vi "Helper - ToggleOverrides.vi"(7 "FocusObj":refnum<vi>, 8 "Rudder Override?":bool, 9 "Sail Override?":bool, 10 "VKey":T1=enum."Up", 11 "Char":i16) -> (1 "Override Rudder":bool, 2 "Override Sail":bool)   [LabVIEW 2011]
doc: "Takes in current values of sail and rudder override and togges them if the correct button is hit.\nOnly does something if you're actually looking at the OCU - use the event structure to get FocusObj.\n\nPotential problem: if you hit the button on the OCU and the keyboard button at the same time, they might end up cancelling each other out....\n\n-Elizabeth Mahon"
uses:
  <vilib>/event_ctls.llb/eventvkey.ctl
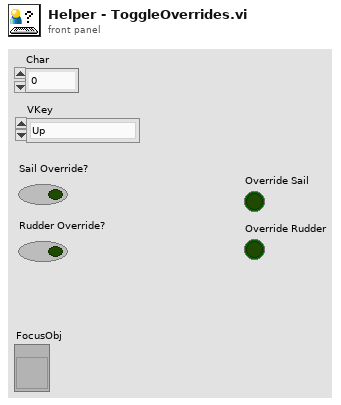
[diagram p1: front panel]
types:
  T1 = typedef "eventvkey.ctl" = enum16{"ASCII", "Enter", "Return", "Shift", "Ctrl", "Alt", "Cmd", "Opt", "Caps", "NumLock", "Clear", "Break", "Up", "Down", "Left", "Right", "Insert", "Delete", "Home", "End", "PageUp", "PageDown", "Escape", "Help", "Pause", "ScrollLock", "F1", "F2", "F3", "F4", "F5", "F6", "F7", "F8", "F9", "F10", "F11", "F12", "F13", "F14", "F15", "F16", "F17", "F18", "F19", "F20", "F21", "F22", "F23", "F24", "Play", "VolumeUp", "VolumeDown", "Mute", "Two Byte Char"}
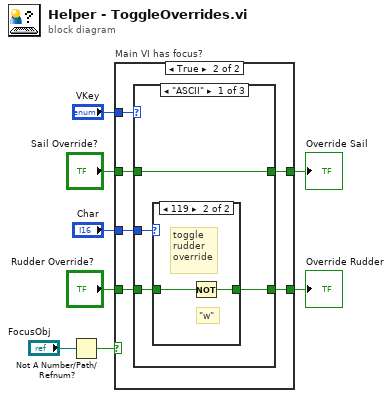
[diagram p0: block diagram]
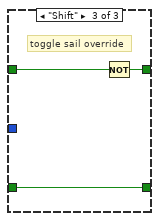
[diagram p5: hidden frame]
diagram:
  n1 = Not A Number/Path/Refnum?(number/path/refnum="FocusObj") -> (NaN/Path/Refnum?=w5:bool)
  n2 = case "Main VI has focus?" shown="True" w5 {
    tunnel: "VKey" -> [_ w16]
    tunnel: "Char" -> [_ w15]
    tunnel: "Sail Override?" -> [w10 w14]
    tunnel: [w10 w13] -> w3
    tunnel: "Rudder Override?" -> [w9 w12]
    tunnel: [w9 w11] -> w1
    frame False {
    }
    frame True {
      n3 = case shown="\"ASCII\"" w16 {
        tunnel: w15 -> [w20 _ _]
        tunnel: w14 -> [w19 w25 w27]
        tunnel: [w19 w25 w28] -> w13
        tunnel: w12 -> [w18 w24 w26]
        tunnel: [w17 w24 w26] -> w11
        frame "ASCII" {
          n4 = case shown="119" w20 {
            tunnel: w18 -> [w21 w23]
            tunnel: [w21 w22] -> w17
            frame 0, Default {
            }
            frame 119 {
              # "toggle\nrudder\noverride"
              # "\"w\""
              n5 = Not(x=w23) -> (.not. x?=w22:bool)
            }
          }
        }
        frame Default {
        }
        frame "Shift" {
          # "toggle sail override"
          n6 = Not(x=w27) -> (.not. x?=w28:bool)
        }
      }
    }
  }
  "Override Sail" <- w3
  "Override Rudder" <- w1
